vi "Read FIFOs.vi"(7 "Mode":T1, 8 "error in (no error)":errorcluster, 11 "RT Data in":T2 {"Label Transfer Config"."Block Data Refs"."Data Reference" format="%.0x"; "Status Config"."HWOut Dur Ref" format="%.0x"; "Status Config"."HWIn Dur Ref" format="%.0x"; "Status Config"."HWOut Count Ref" format="%.0x"; "Status Config"."HWIn Count Ref" format="%.0x"; "Status Config"."Error Data Ref" format="%.0x"; "HWOutput Channels"."Labels Settings"."Driver Data"."Num Bits" min=1 max=32; "HWOutput Channels"."Labels Settings"."Driver Data"."Start Bit" min=8 max=31; "HWOutput Channels"."Labels Settings"."Block Data Refs"."Data Reference" format="%.0x"; "HWOutput Channels"."Labels Settings"."Label" format="%.0o"; "HWInput Channels"."Labels Settings"."Driver Data"."Num Bits" min=1 max=32; "HWInput Channels"."Labels Settings"."Driver Data"."Start Bit" min=8 max=31; "HWInput Channels"."Labels Settings"."Block Data Refs"."Data Reference" format="%.0x"; "HWInput Channels"."Labels Settings"."Label" format="%.0o"}) -> (0 "error out":errorcluster, 3 "RT Data out":T2 {"Label Transfer Config"."Block Data Refs"."Data Reference" format="%.0x"; "Status Config"."HWOut Dur Ref" format="%.0x"; "Status Config"."HWIn Dur Ref" format="%.0x"; "Status Config"."HWOut Count Ref" format="%.0x"; "Status Config"."HWIn Count Ref" format="%.0x"; "Status Config"."Error Data Ref" format="%.0x"; "HWOutput Channels"."Labels Settings"."Driver Data"."Num Bits" min=1 max=32; "HWOutput Channels"."Labels Settings"."Driver Data"."Start Bit" min=8 max=31; "HWOutput Channels"."Labels Settings"."Block Data Refs"."Data Reference" format="%.0x"; "HWOutput Channels"."Labels Settings"."Label" format="%.0o"; "HWInput Channels"."Labels Settings"."Driver Data"."Num Bits" min=1 max=32; "HWInput Channels"."Labels Settings"."Driver Data"."Start Bit" min=8 max=31; "HWInput Channels"."Labels Settings"."Block Data Refs"."Data Reference" format="%.0x"; "HWInput Channels"."Labels Settings"."Label" format="%.0o"})   [LabVIEW 2011, in "AIT 1553 Custom Device.lvlib"]
uses:
  AIT 1553 Custom Device.lvlib
  RT Controls/RT Data.ctl
  RT Controls/RT HW Channel.ctl
  RT Controls/RT Label Settings.ctl
  Controls and Global/Label.ctl
  Controls and Global/transferPeriod.ctl
  <vilib>/NI Veristand/Custom Device API/Block Data Reference.ctl
  <vilib>/NI Veristand/Custom Device API/Data Reference.ctl
  RT Controls/Driver Data.ctl
  Controls and Global/Start Bit.ctl
  Controls and Global/Number of Bits.ctl
  RT Controls/Error Qs.ctl
  RT Controls/Status Channels Config.ctl
  RT Controls/FIFO.ctl
  RT Controls/Label Transfer Config.ctl
  <userlib>/ARINC-429/vi/enum/Owl429HardwareSource.ctl
  RT Controls/ReadWrite Selector.ctl
  <vilib>/NI Veristand/Custom Device API/Custom Device API.lvlib
  <userlib>/ARINC-429/Owl429.lvlib
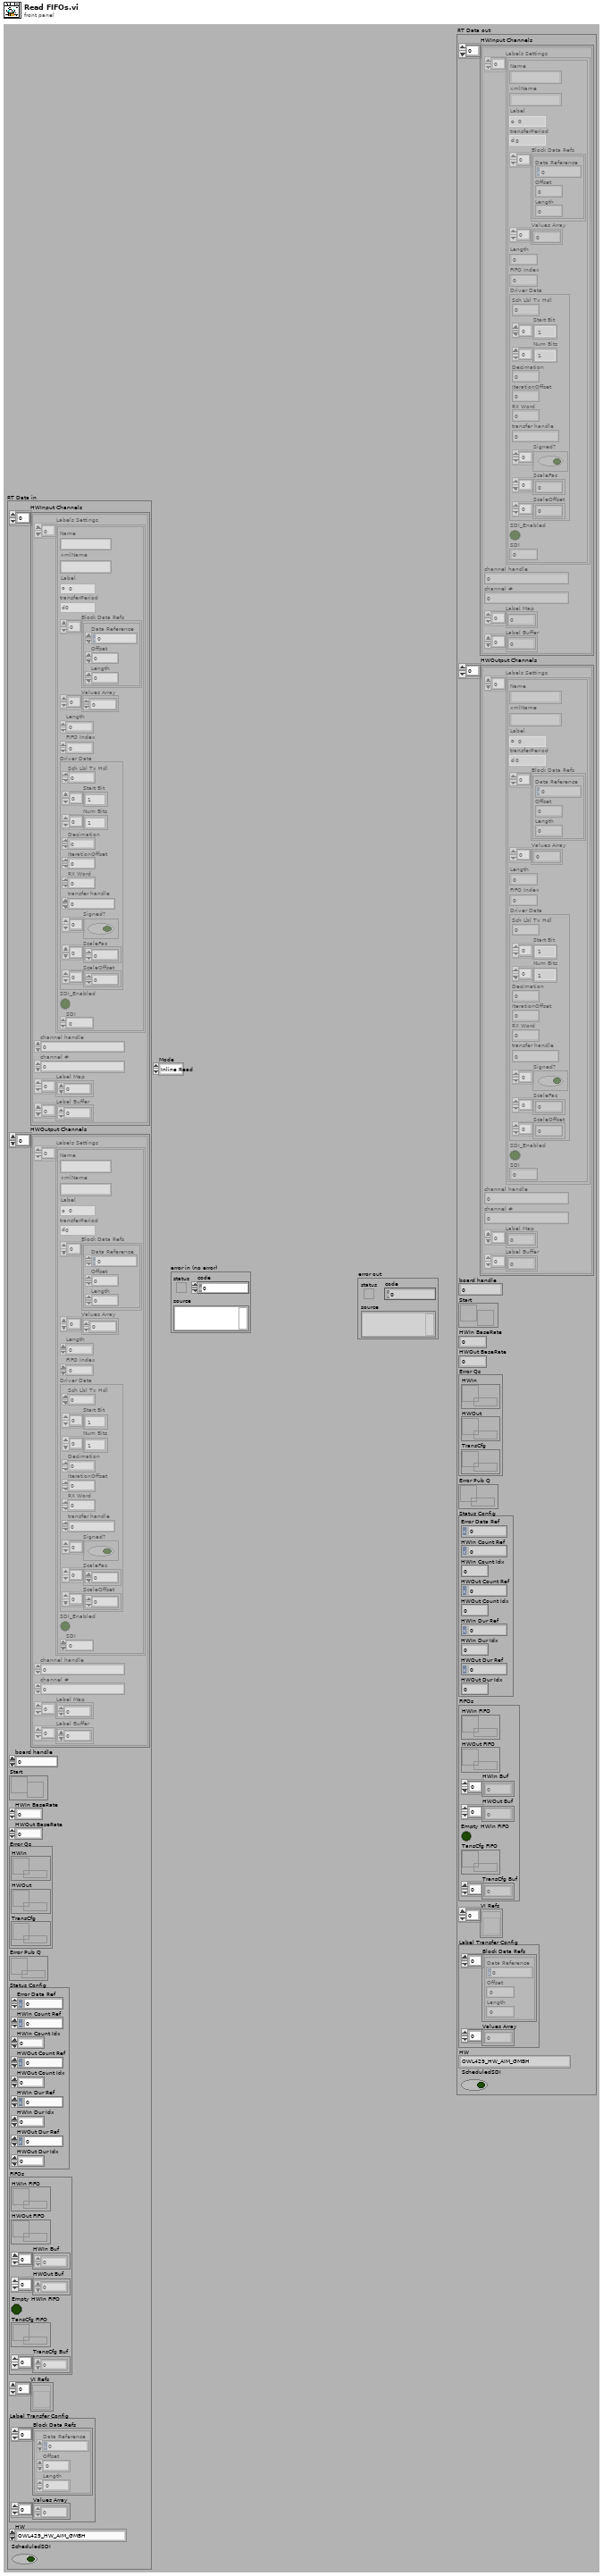
[diagram p1: front panel]
types:
  T1 = typedef "AIT 1553 Custom Device.lvlib/ReadWrite Selector.ctl" = enum16{"Inline Read", "Inline Write", "Async HWIn", "Async HWOut"}
  T2 = typedef "AIT 1553 Custom Device.lvlib/RT Data.ctl" = cluster{"HWInput Channels":T3[], "HWOutput Channels":T3[], "board handle":u32, "Start":refnum<notifier>, "HWIn BaseRate":i64, "HWOut BaseRate":i64, "Error Qs":T12, "Error Pub Q":refnum<queue>, "Status Config":T13, "FIFOs":T14, "VI Refs":refnum<vi>[], "Label Transfer Config":T15, "HW":T16, "ScheduledSDI":bool}
  T3 = typedef "AIT 1553 Custom Device.lvlib/RT HW Channel.ctl" = cluster{"Labels Settings":T4[], "channel handle":u32, "channel #":u16, "Label Map":i32[], "Label Buffer":u32[]}
  T4 = typedef "AIT 1553 Custom Device.lvlib/RT Label Settings.ctl" = cluster{"Name":string, "xmlName":string, "Label":T5, "transferPeriod":T6, "Block Data Refs":T7[], "Values Array":dbl[], "Length":i32, "FIFO Index":i32, "Driver Data":T9, "SDI_Enabled":bool, "SDI":u8}
  T5 = typedef "AIT 1553 Custom Device.lvlib/Label.ctl" = u8
  T6 = typedef "AIT 1553 Custom Device.lvlib/transferPeriod.ctl" = u32
  T7 = typedef "Custom Device API.lvlib/Block Data Reference.ctl" = cluster{"Data Reference":T8, "Offset":i32, "Length":i32}
  T8 = typedef "Custom Device API.lvlib/Data Reference.ctl" = i32
  T9 = typedef "AIT 1553 Custom Device.lvlib/Driver Data.ctl" = cluster{"Sch Lbl Tx Hdl":u32, "Start Bit":T10[], "Num Bits":T11[], "Decimation":i32, "IterationOffset":i32, "RX Word":u32, "transfer handle":u32, "Signed?":bool[], "ScaleFac":dbl[], "ScaleOffset":dbl[]}
  T10 = typedef "AIT 1553 Custom Device.lvlib/Start Bit.ctl" = i32
  T11 = typedef "AIT 1553 Custom Device.lvlib/Number of Bits.ctl" = i32
  T12 = typedef "AIT 1553 Custom Device.lvlib/Error Qs.ctl" = cluster{"HWIn":refnum<queue>, "HWOut":refnum<queue>, "TransCfg":refnum<queue>}
  T13 = typedef "AIT 1553 Custom Device.lvlib/Status Channels Config.ctl" = cluster{"Error Data Ref":T8, "HWIn Count Ref":T8, "HWIn Count Idx":i32, "HWOut Count Ref":T8, "HWOut Count Idx":i32, "HWIn Dur Ref":T8, "HWIn Dur Idx":i32, "HWOut Dur Ref":T8, "HWOut Dur Idx":i32}
  T14 = typedef "AIT 1553 Custom Device.lvlib/FIFO.ctl" = cluster{"HWIn FIFO":refnum<k33>, "HWOut FIFO":refnum<k33>, "HWIn Buf":dbl[], "HWOut Buf":dbl[], "Empty HWIn FIFO":bool, "TansCfg FIFO":refnum<k33>, "TransCfg Buf":dbl[]}
  T15 = typedef "AIT 1553 Custom Device.lvlib/Label Transfer Config.ctl" = cluster{"Block Data Refs":T7[], "Values Array":dbl[]}
  T16 = typedef "Owl429.lvlib/Owl429HardwareSource.ctl" = enum16{"OWL429_HW_AIM_GMBH", "OWL429_HW_AIT"}
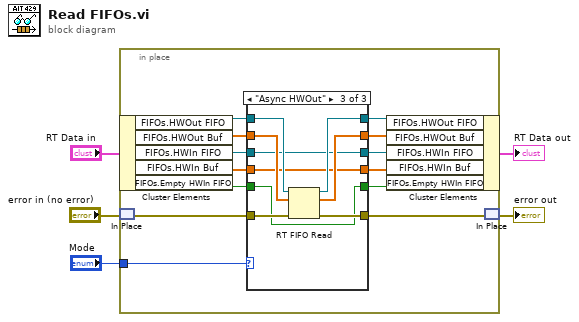
[diagram p0: block diagram]
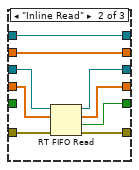
[diagram p3: hidden frame]
diagram:
  n1 = in-place {
    in-place-border: "Mode" -> [w11]
    n2 = in-place-cluster #1("RT Data in") -> ("FIFOs.HWOut FIFO"=w9:refnum<k33>, "FIFOs.HWOut Buf"=w8:dbl[], "FIFOs.HWIn FIFO"=w18:refnum<k33>, "FIFOs.HWIn Buf"=w17:dbl[], "FIFOs.Empty HWIn FIFO"=w10:bool)
    n3 = in-place-match #2("error in (no error)") -> (w13:errorcluster)
    n4 = case shown="\"Async HWOut\"" w11 {
      tunnel: w18 -> [w23 w33 w35]
      tunnel: w17 -> [w24 w32 w36]
      tunnel: [w24 w31 w36] -> w16
      tunnel: [w23 w30 w35] -> w15
      tunnel: [w22 w29 w34] -> w14
      tunnel: w13 -> [w21 w28 w42]
      tunnel: [w21 w27 w41] -> w12
      tunnel: w10 -> [w22 _ w34]
      tunnel: w9 -> [w19 w25 w40]
      tunnel: w8 -> [w20 w26 w39]
      tunnel: [w19 w25 w38] -> w7
      tunnel: [w20 w26 w37] -> w6
      frame Default {
      }
      frame "Inline Read" {
        n5 = RT FIFO Read(0:w33, 1:w32, 3:w28) -> (8:w30:refnum<k33>, 9:w31:dbl[], 10:w29:bool, 11:w27:errorcluster)  [unwired: 1 in, 1 out]
      }
      frame "Async HWOut" {
        n6 = RT FIFO Read(0:w40, 1:w39, 3:w42) -> (8:w38:refnum<k33>, 9:w37:dbl[], 11:w41:errorcluster)  [unwired: 1 in, 2 out]
      }
    }
    n7 = in-place-cluster #1("FIFOs.HWOut FIFO"=w7, "FIFOs.HWOut Buf"=w6, "FIFOs.HWIn FIFO"=w15, "FIFOs.HWIn Buf"=w16, "FIFOs.Empty HWIn FIFO"=w14) -> (→"RT Data out":T2)
    n8 = in-place-match #2(w12) -> (→"error out":errorcluster)
  }
